vi "Do.vi"(8 "error in (no error)":errorcluster, 10 "Actor in":refnum<class "Actor.lvclass">, 11 "Update Error Msg in":refnum<class "Update Error Msg.lvclass">) -> (0 "error out":errorcluster, 2 "Actor out":refnum<class "Actor.lvclass">)   [LabVIEW 2016, in "Example Actor.lvlib" / "Update Error Msg.lvclass"]
doc: "(<B>Filename</B>: Actor Framework.lvlib:Message.lvclass:Do.vi)\n\nDefines what a message does when it is received by an actor. Generally, a message instructs an actor to invoke one of its methods. By default, this method does nothing. A child class must override it to define behavior. Create a child class by using the Actor Framework Message Maker dialog box."
uses:
  Update Error Msg.lvclass
  C:/Project/Shared Libraries/Iterator Actor/Iterator Actor 2/Iterator Report Error Msg/Iterator Report Error Msg.lvclass
  <vilib>/ActorFramework/Actor/Actor.lvclass
  Example Actor/Example Actor.lvclass
  C:/Program Files (x86)/National Instruments/LabVIEW 2016/vi.lib/ActorFramework/Actor/Actor.lvclass
  Iterator Actor/Iterator Actor Abstract Messages/Iterator Report Error Msg/Iterator Report Error Msg.lvclass
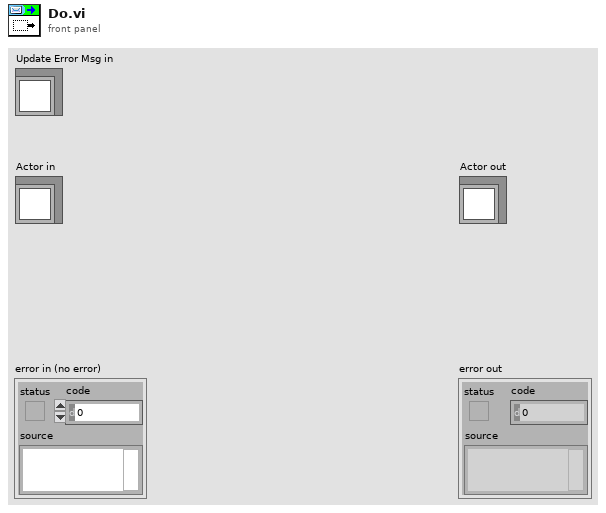
[diagram p1: front panel]
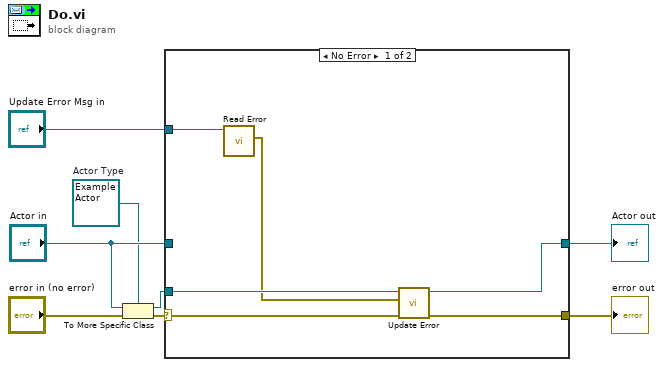
[diagram p0: block diagram]
diagram:
  w3 = refnum<class "Example Actor.lvclass"> refnum  # Actor Type
  n1 = To More Specific Class(target class=w3, reference="Actor in", error in="error in (no error)") -> (specific class reference=w2:refnum<class "Example Actor.lvclass">, error out=w7:errorcluster)
  n2 = case shown="No Error" w7 {
    selector: w7 -> [w12 w16]
    tunnel: [w14 w16] -> w6
    tunnel: [w13 w15] -> w5
    tunnel: "Actor in" -> [_ w15]
    tunnel: w2 -> [w11 _]
    tunnel: "Update Error Msg in" -> [w10 _]
    frame No Error {
      n3 = call "Read Error.vi"("Iterator Report Error Msg"=w10) -> ("Error"=w9:errorcluster)  [unwired: 10 in]
      n4 = call "Update Error.vi"("error in (no error)"=w12, "Received Error"=w9, "Example Actor in"=w11) -> ("error out"=w14:errorcluster, "Example Actor out"=w13:refnum<class "Example Actor.lvclass">)  [unwired: 7 in]
    }
    frame Error {
    }
  }
  "error out" <- w6
  "Actor out" <- w5
